vi "Read stop event.vi"(8 "error in (no error)":errorcluster, 11 "Mag Lab Root in":refnum<class "Mag Lab Root.lvclass">) -> (0 "error out":errorcluster, 2 "stop event":refnum<user-event>, 3 "Mag Lab Root out":refnum<class "Mag Lab Root.lvclass">)   [LabVIEW 2015, in "Mag Lab Root.lvclass"]
uses:
  Mag Lab Root.lvclass
  Mag Lab Root.lvclass/Mag Lab Root.ctl
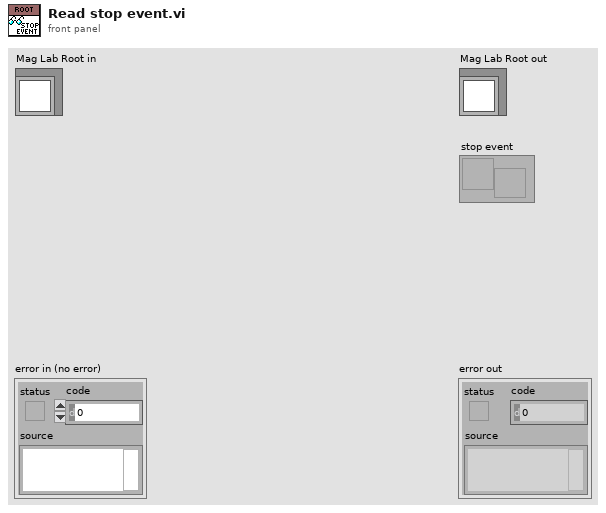
[diagram p1: front panel]
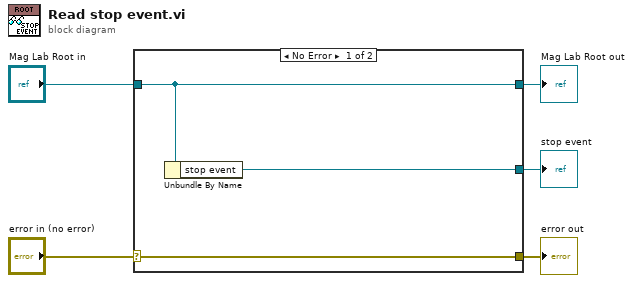
[diagram p0: block diagram]
diagram:
  n1 = case shown="No Error" "error in (no error)" {
    selector: "error in (no error)" -> [w8 w9]
    tunnel: [w8 w9] -> w4
    tunnel: [w7 w10] -> w2
    tunnel: "Mag Lab Root in" -> [w7 w10]
    tunnel: [w6 _] -> w1
    frame No Error {
      n2 = Unbundle By Name(w7) -> ("stop event"=w6:refnum<user-event>)
    }
    frame Error {
    }
  }
  "error out" <- w4
  "Mag Lab Root out" <- w2
  "stop event" <- w1
